vi "test.vi"() -> ()   [LabVIEW 2014]
panel:
  out "element 2":u32
  out "element":u32
  out "size(s)":i32
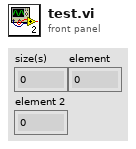
[diagram p1: front panel]
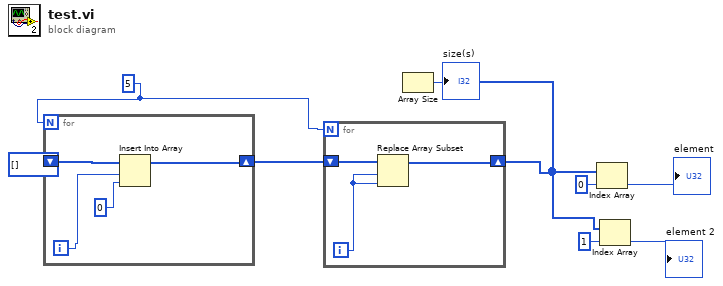
[diagram p0: block diagram]
diagram:
  w1 = 5
  n1 = for {
    N: w1 -> [_]
    shift-right: [w12] -> w3
    shift-left: u32[] [] ("array") -> [w13]
    i -> [w11]
    n2 = Insert Into Array(array=w13, index=w11, new element=u32 0 ("new element/subarray")) -> (w12:u32[])
  }
  n3 = for {
    N: w1 -> [_]
    shift-right: [w14] -> w2
    shift-left: w3 -> [w16]
    i -> [w15]
    n4 = Replace Array Subset "Replace Array Subset"(array=w16, new element=w15, index=w15) -> (w14:u32[])
  }
  n5 = Array Size(array=w2) -> (size(s)=→"size(s)":i32)
  n6 = Index Array(array=w2, index=0) -> (element=→"element":u32)
  n7 = Index Array(array=w2, index=1) -> (element=→"element 2":u32)
